vi "init Compressor.vi"(1 "error in (no error)":errorcluster) -> (0 "error out":errorcluster)   [LabVIEW 2020]
uses:
  <vilib>/Rock Robotics/WPI/Utilities/WPI_GetSetVariantRefNum.vi
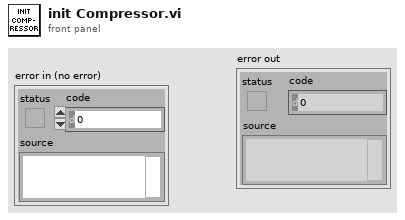
[diagram p1: front panel]
types:
  T1 = typedef "WPI_CompressorDevRef.ctl" = cluster{"DevStatus":errorcluster, "Pneumatics Control Module":u8}
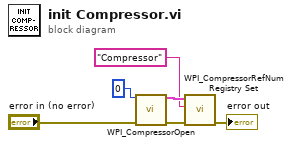
[diagram p0: block diagram]
diagram:
  n1 = call <vilib>:"WPI_CompressorOpen.vi"("Pneumatics device (def)"=u8 0, "error in (no error)"="error in (no error)") -> ("CompressorDevRef"=w6:T1, "error out"=w3:errorcluster)  [unwired: 12 in]
  n2 = call <vilib>:"WPI_CompressorRefNum Registry Set.vi"("error in (no error)"=w3, "refnum name"="Compressor", "CompressorDevRef"=w6) -> ("error out"=→"error out":errorcluster)  [unwired: 7 in, 1 out]
